vi "Configure Measurement (Demodulation).vi"(0 "VISA resource name":refnum<visa-resource-name>, 1 "Carrier Frequency Step (1E+8 Hz)":dbl=100000000.0, 5 "Auto Carrier Frequency (F: Disable)":bool, 9 "Carrier Frequency (2.5E+6 Hz)":dbl=2500000.0, 11 "error in (no error)":errorcluster, 12 "External Gain (0 dB)":dbl) -> (4 "VISA resource name out":refnum<visa-resource-name>, 15 "error out":errorcluster)   [LabVIEW 2022 SP3, in "Agilent N934X Series.lvlib"]
doc: "Configures the general setting of Demodulation Option.\n\nNote:\nThis VI is only applicable for N9321C, N9322C, N9323C, N9324C models"
uses:
  <instrlib>/Agilent N934X Series/Agilent N934X Series.lvlib
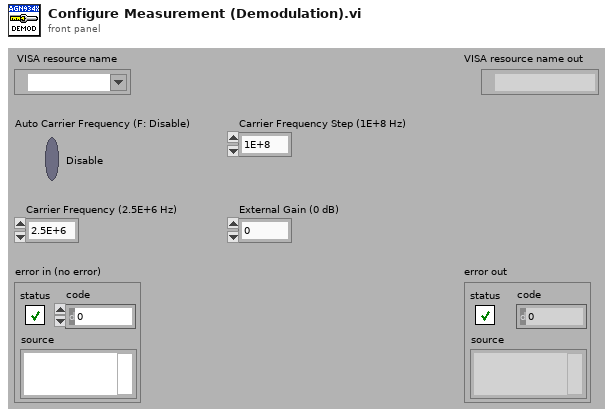
[diagram p1: front panel]
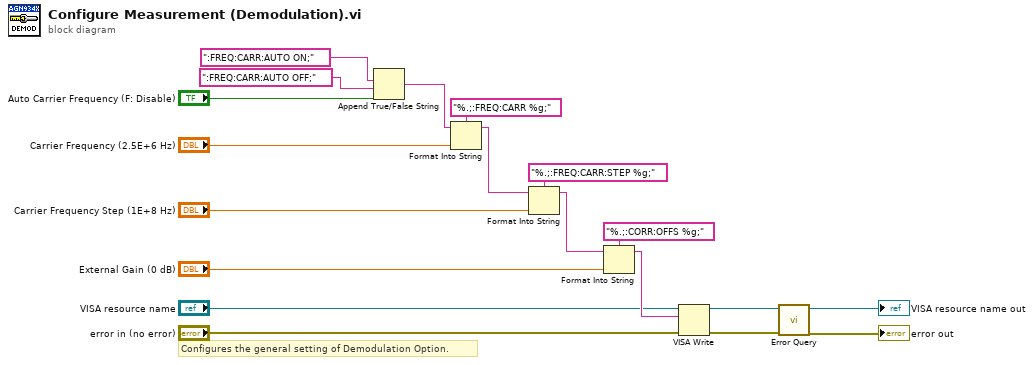
[diagram p0: block diagram]
diagram:
  # "Configures the general setting of Demodulation Option."
  n1 = Append True/False String(1:"Auto Carrier Frequency (F: Disable)", 2:":FREQ:CARR:AUTO OFF;", 3:":FREQ:CARR:AUTO ON;") -> (0:w2:string)  [unwired: 1 in]
  n2 = Format Into String(format string="%.;:FREQ:CARR %g;", initial string=w2, "Carrier Frequency (2.5E+6 Hz)") -> (resulting string=w1:string)  [unwired: 1 in, 1 out]
  n3 = Format Into String(format string="%.;:FREQ:CARR:STEP %g;", initial string=w1, "Carrier Frequency Step (1E+8 Hz)") -> (resulting string=w12:string)  [unwired: 1 in, 1 out]
  n4 = Format Into String(format string="%.;:CORR:OFFS %g;", initial string=w12, "External Gain (0 dB)") -> (resulting string=w9:string)  [unwired: 1 in, 1 out]
  n5 = VISA Write(VISA resource name="VISA resource name", write buffer=w9, error in (no error)="error in (no error)") -> (VISA resource name out=w6:refnum<visa-resource-name>, error out=w5:errorcluster)  [unwired: 1 out]
  n6 = call <instrlib>:"Error Query.vi"("error in (no error)"=w5, "VISA resource name"=w6) -> ("error out"=→"error out":errorcluster, "VISA resource name out"=→"VISA resource name out":refnum<visa-resource-name>)  [unwired: 6 in, 2 out]
